vi "Write Mandatory Sleep.vi"(8 "error in (no error)":errorcluster, 10 "Mandatory Sleep":u32 format="%d us", 11 "Simulated VeriStand Engine in":refnum<class "Simulated VeriStand Engine.lvclass">) -> (0 "error out":errorcluster, 3 "Simulated VeriStand Engine out":refnum<class "Simulated VeriStand Engine.lvclass">)   [LabVIEW 2016, in "Simulated VeriStand Engine.lvclass"]
uses:
  Simulated VeriStand Engine.lvclass
  Simulated VeriStand Engine.lvclass/Simulated VeriStand Engine.ctl
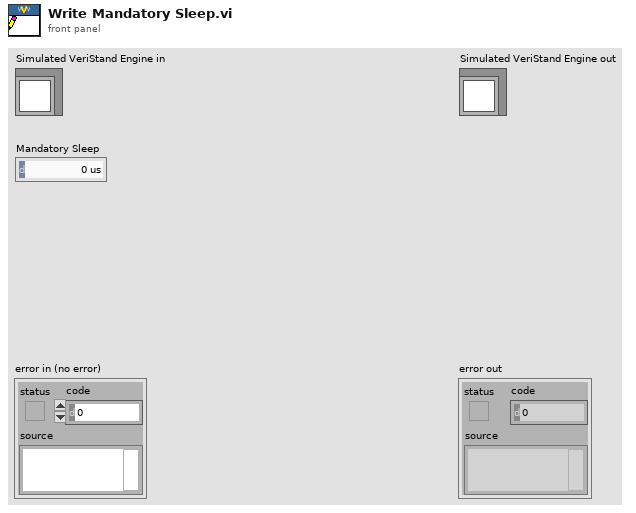
[diagram p1: front panel]
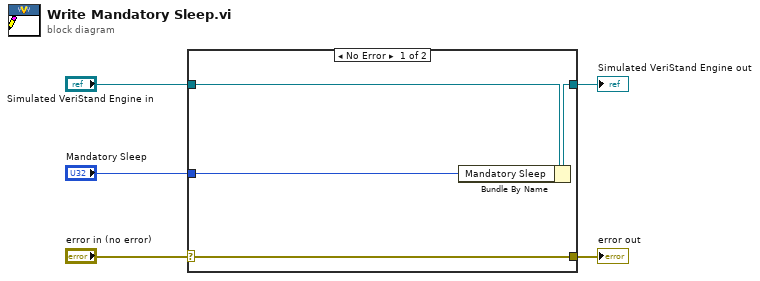
[diagram p0: block diagram]
diagram:
  n1 = case shown="No Error" "error in (no error)" {
    selector: "error in (no error)" -> [w9 w10]
    tunnel: [w9 w10] -> w4
    tunnel: [w7 w11] -> w2
    tunnel: "Simulated VeriStand Engine in" -> [w8 w11]
    tunnel: "Mandatory Sleep" -> [w6 _]
    frame No Error {
      n2 = Bundle By Name(cluster=w8, "Mandatory Sleep"=w6) -> (w7:refnum<class "Simulated VeriStand Engine.lvclass">)
    }
    frame Error {
    }
  }
  "error out" <- w4
  "Simulated VeriStand Engine out" <- w2
